vi "VI_ReadData.vi"(8 "error in (no error)":errorcluster, 10 "Common Refs":T1, 11 "queue":refnum<queue>) -> (0 "error out":errorcluster)   [LabVIEW 2020]
uses:
  TypeDefs/Refs_Common.ctl
  <vilib>/Stadlmann TEC/OXYGEN Datastream/VIs/Data Aquasation/TypeDefs/DataPoint_Double.ctl
  <vilib>/Stadlmann TEC/OXYGEN Datastream/VIs/Data Aquasation/SubVIs/GetDataPackage_Double.vi
  <vilib>/Stadlmann TEC/OXYGEN Datastream/OXYGEN_Datastream.lvlib
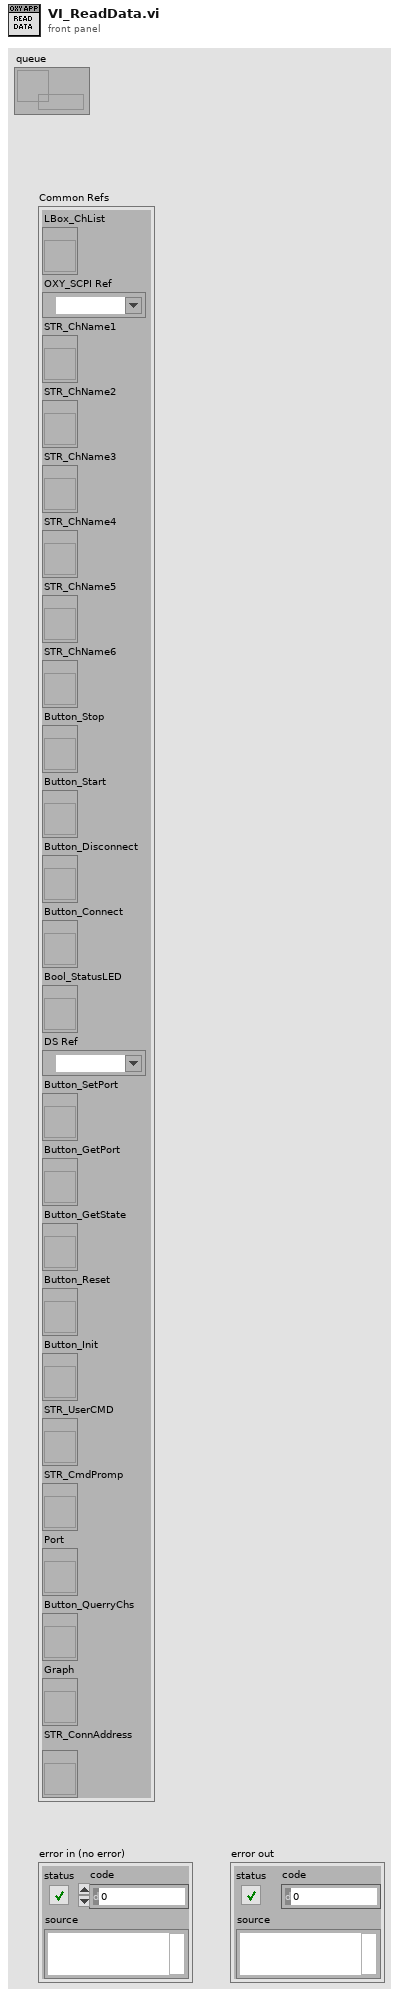
[diagram p1: front panel]
types:
  T1 = typedef "Refs_Common.ctl" = cluster{"LBox_ChList":refnum<vi>, "OXY_SCPI Ref":refnum<visa-resource-name>, "STR_ChName1":refnum<vi>, "STR_ChName2":refnum<vi>, "STR_ChName3":refnum<vi>, "STR_ChName4":refnum<vi>, "STR_ChName5":refnum<vi>, "STR_ChName6":refnum<vi>, "Button_Stop":refnum<vi>, "Button_Start":refnum<vi>, "Button_Disconnect":refnum<vi>, "Button_Connect":refnum<vi>, "Bool_StatusLED":refnum<vi>, "DS Ref":refnum<visa-resource-name>, "Button_SetPort":refnum<vi>, "Button_GetPort":refnum<vi>, "Button_GetState":refnum<vi>, "Button_Reset":refnum<vi>, "Button_Init":refnum<vi>, "STR_UserCMD":refnum<vi>, "STR_CmdPromp":refnum<vi>, "Port":refnum<vi>, "Button_QuerryChs":refnum<vi>, "Graph":refnum<vi>, "STR_ConnAddress":refnum<vi>}
  T2 = typedef "OXYGEN_Datastream.lvlib/DataPoint_Double.ctl" = cluster{"DataPoints":cluster{"Time":dbl, "Value":dbl}[]}
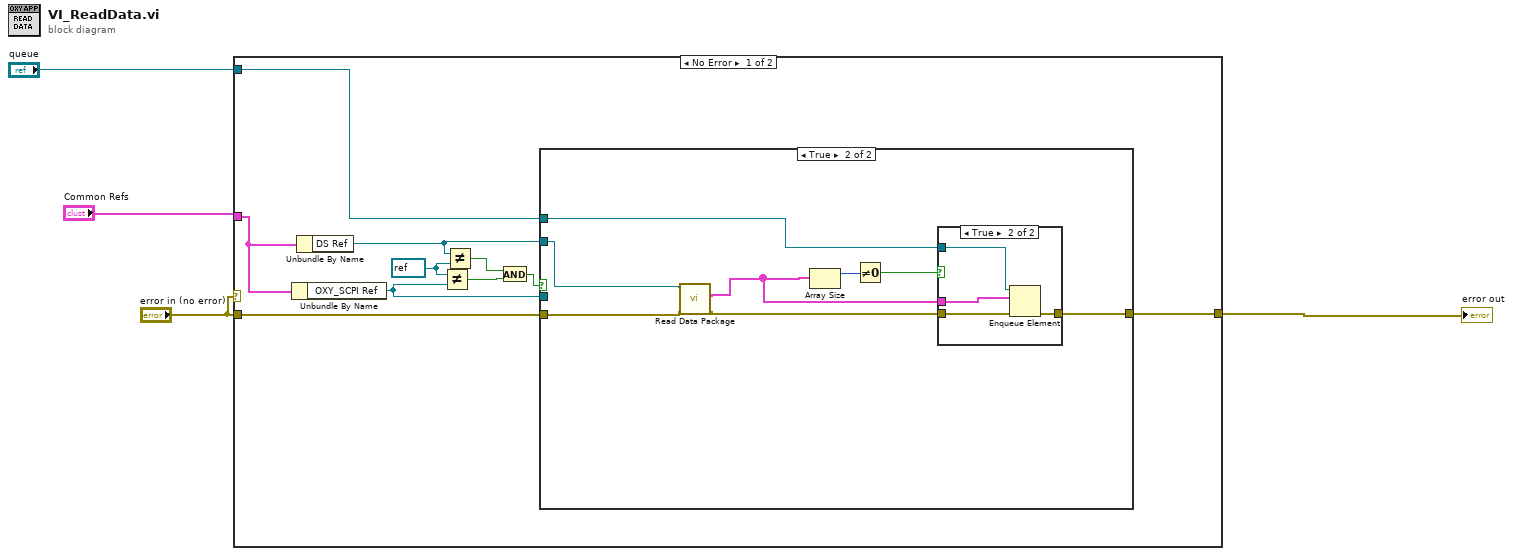
[diagram p0: block diagram]
diagram:
  n1 = case shown="No Error" "error in (no error)" {
    tunnel: [w14 w29] -> w4
    tunnel: "error in (no error)" -> [w10 w29]
    tunnel: "queue" -> [w8 _]
    tunnel: "Common Refs" -> [w5 _]
    frame No Error {
      w11 = refnum<visa-resource-name> refnum ("OXY_SCPI Ref")
      n2 = Unbundle By Name(w5) -> ("OXY_SCPI Ref"=w13:refnum<visa-resource-name>)
      n3 = Unbundle By Name(w5) -> ("DS Ref"=w9:refnum<visa-resource-name>)
      n4 = Not Equal?(x=w11, y=w13) -> (x != y?=w12:bool)
      n5 = Not Equal?(x=w9, y=w11) -> (x != y?=w6:bool)
      n6 = And(x=w6, y=w12) -> (x .and. y?=w7:bool)
      n7 = case shown="True" w7 {
        tunnel: w8 -> [_ w21]
        tunnel: w9 -> [_ w17]
        tunnel: w10 -> [w15 w16]
        tunnel: w13 -> [_ _]
        tunnel: [w15 w20] -> w14
        frame False {
        }
        frame True {
          n8 = call-poly <vilib>:"Read Data Package.vi"("error in (no error)"=w16, "VISA Refnum in"=w17) -> ("error out"=w19:errorcluster, "Data"=w18:T2[])  [unwired: 6 in, 2 out]
          n9 = Array Size(array=w18) -> (size(s)=w23:i32)
          n10 = Not Equal To 0?(x=w23) -> (x != 0?=w22:bool)
          n11 = case shown="True" w22 {
            tunnel: w21 -> [_ w28]
            tunnel: [w24 w27] -> w20
            tunnel: w19 -> [w24 w25]
            tunnel: w18 -> [_ w26]
            frame False {
            }
            frame True {
              n12 = Enqueue Element(queue=w28, element=w26, error in (no error)=w25) -> (error out=w27:errorcluster)  [unwired: 1 in, 2 out]
            }
          }
        }
      }
    }
    frame Error {
    }
  }
  "error out" <- w4
